vi "FindFilesNotRelativeToProjectRoot.vi"() -> ()   [LabVIEW 2020]
uses:
  <vilib>/Utility/lvfile.llb/NI_FileType.lvlib
  <vilib>/picture/picture.llb/imagedata.ctl
  <userlib>/_OpenG.lib/file/file.llb/openg_file.lvlib
  <userlib>/_OpenG.lib/file/file.llb/Valid Path - Traditional__ogtk.vi
  Microsoft.VisualBasic
panel:
  in  "Project":u16(ring)
  in  "Files Not in Project":i32[](listbox) caption="Files Not in Project (these files are on disk under the top-level project folder, but do not exist anywhere within the project)"
  in  "Move Files":bool
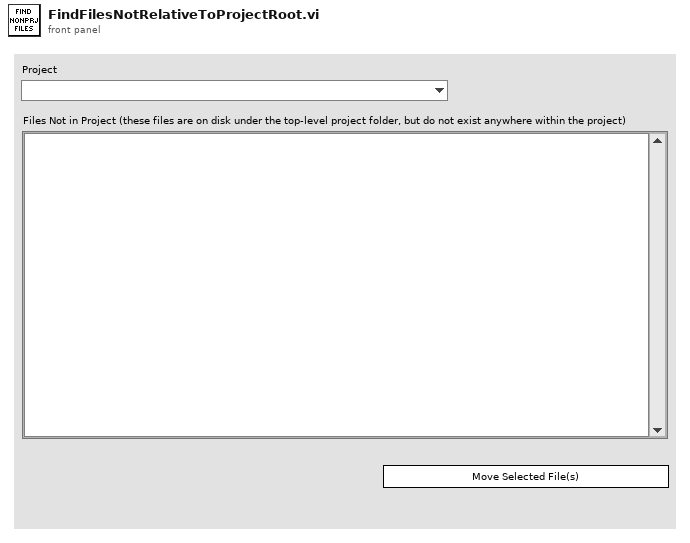
[diagram p1: front panel]
types:
  T1 = enum8{"Enabled", "Disabled", "Disabled and Grayed Out"}
  T2 = typedef "imagedata.ctl" = cluster{"image type":i32, "image depth":i32, "image":u8[], "mask":u8[], "colors":u32[], "Rectangle":cluster{"left":i16, "top":i16, "right":i16, "bottom":i16}}
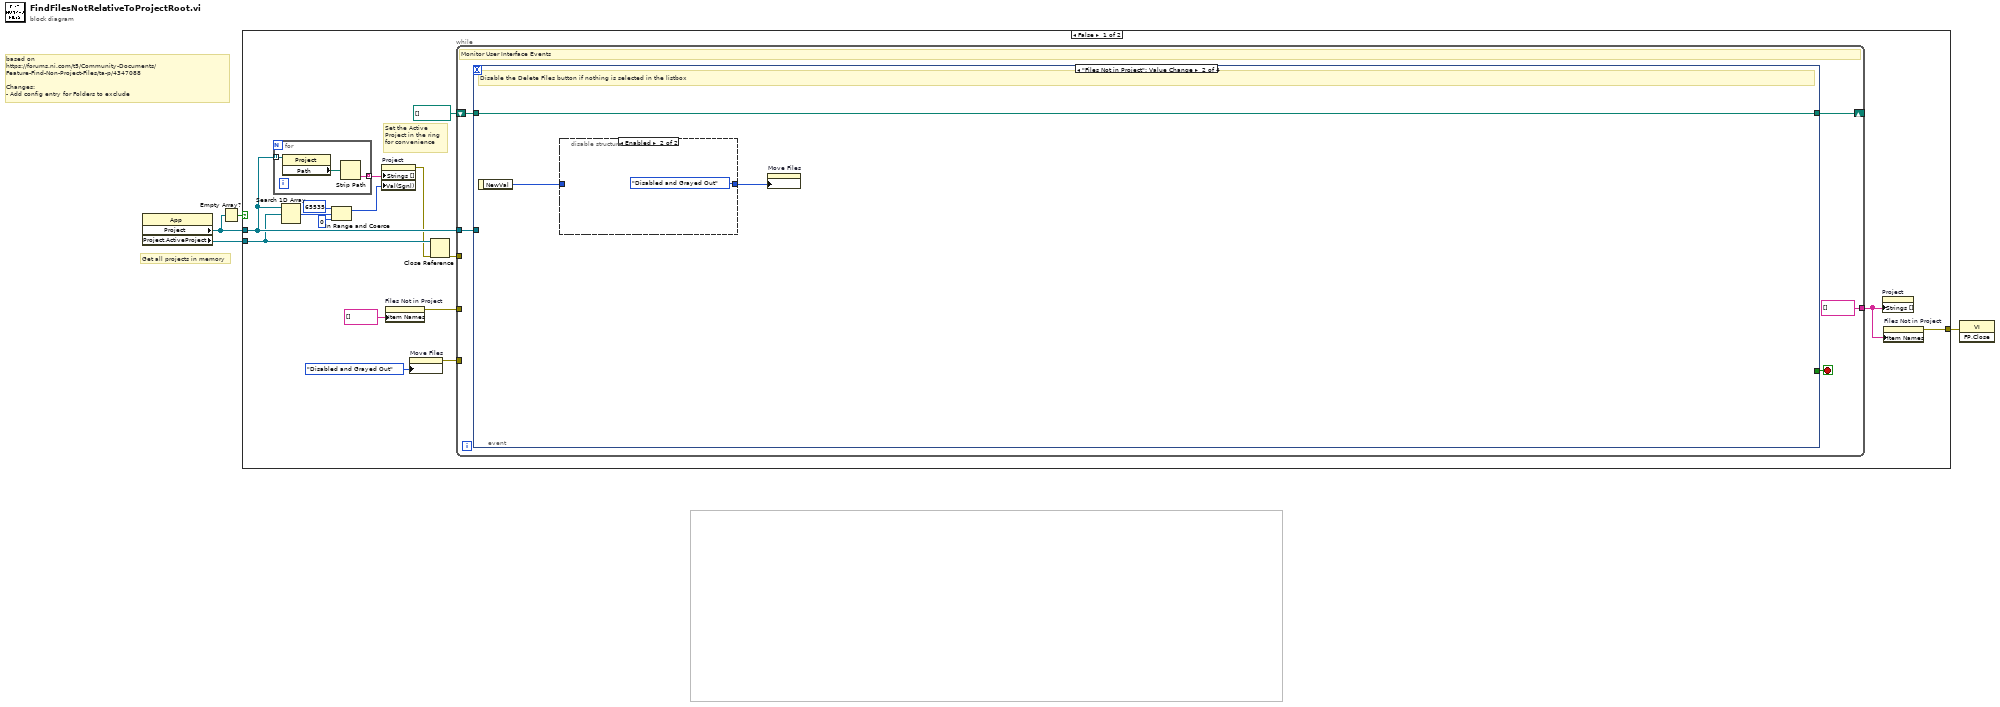
[diagram p0: block diagram]
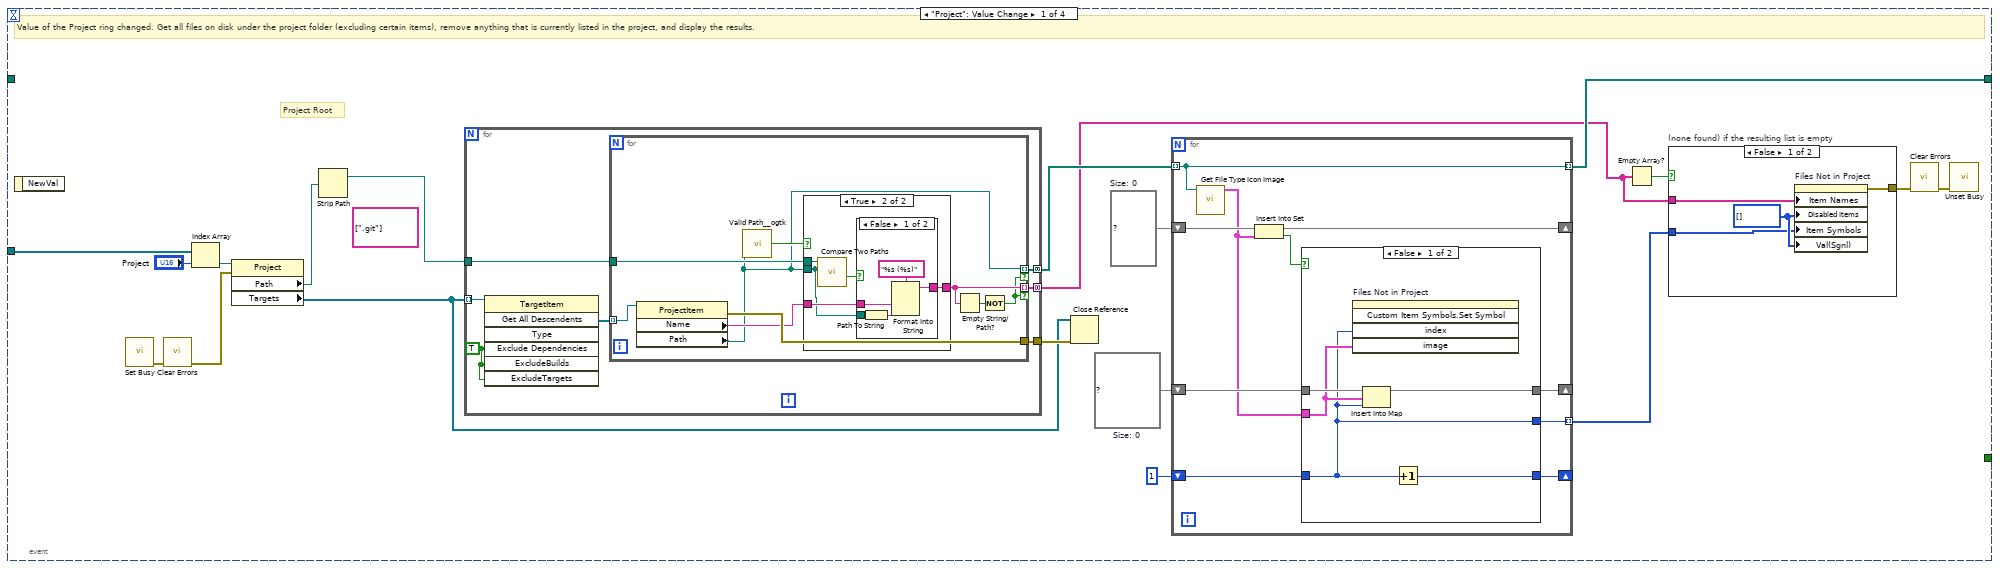
[diagram p2: hidden frame]
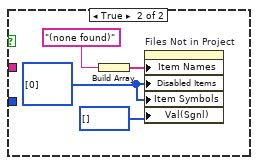
[diagram p3: hidden frame]
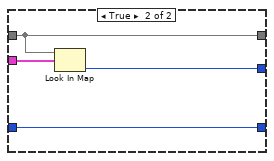
[diagram p6: hidden frame]
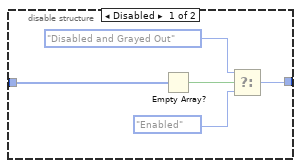
[diagram p7: hidden frame]
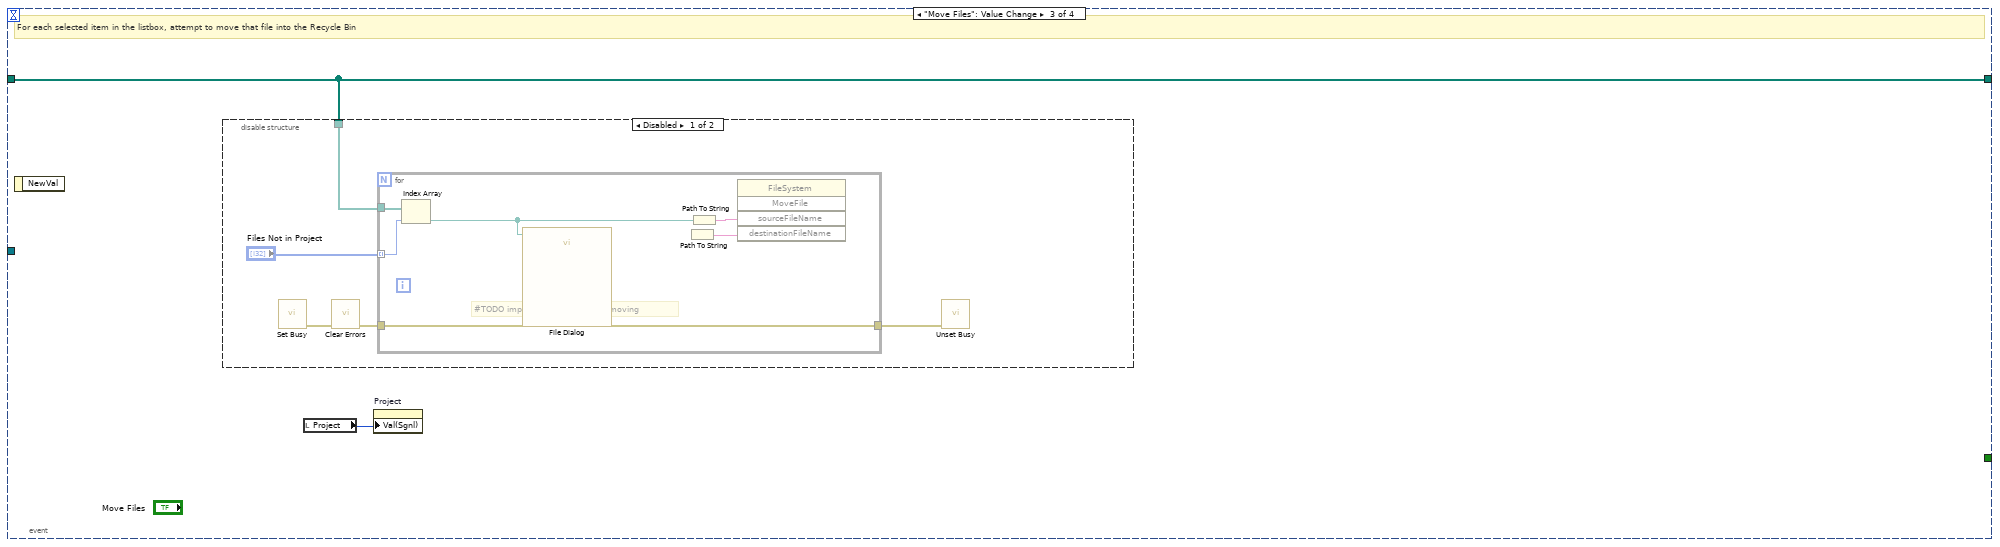
[diagram p8: hidden frame]
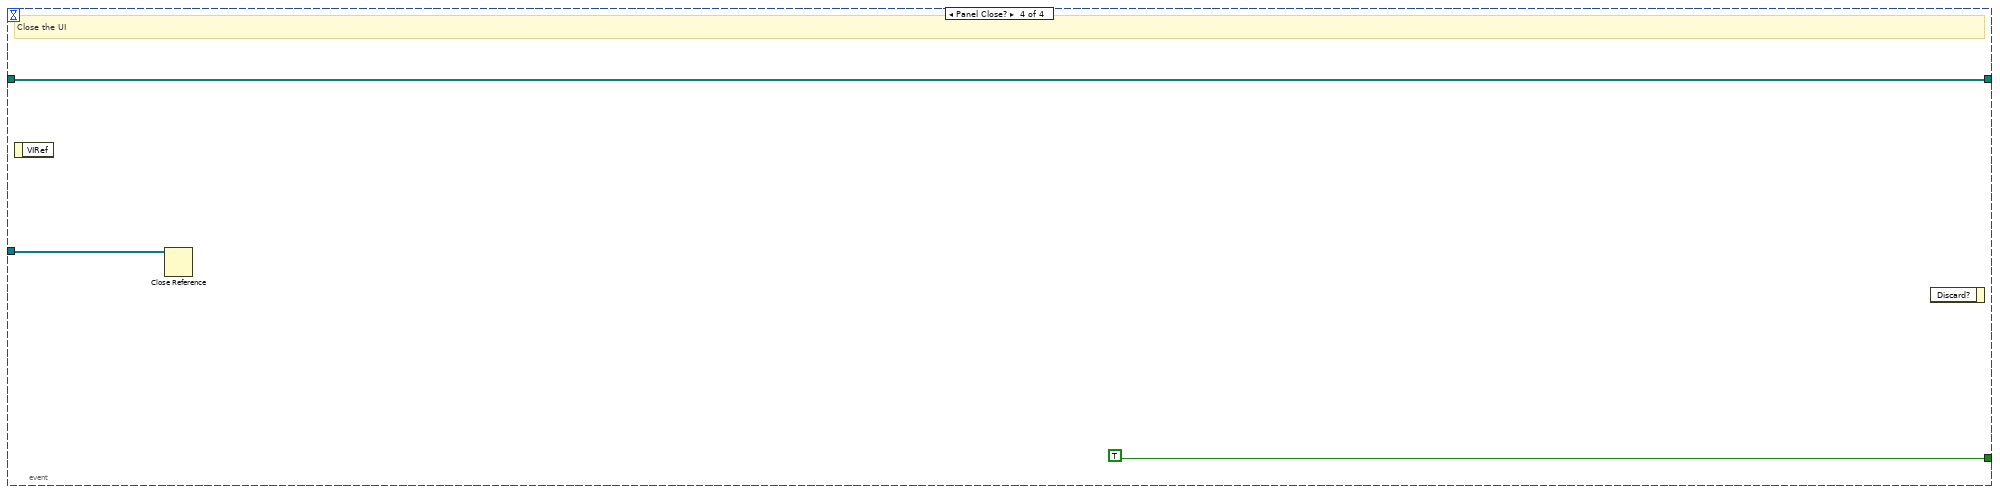
[diagram p10: hidden frame]
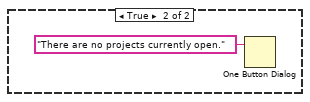
[diagram p11: hidden frame]
diagram:
  # "based on\nhttps://forums.ni.com/t5/Community-Documents/Feature-Find-Non-Project-Files/ta-p/4347088\n\nChanges:\n- Add config entry for Folders to exclude"
  # "Get all projects in memory"
  n1 = property class="App"() -> ("Project"=w3:refnum<vi>[], "Project.ActiveProject"=w4:refnum<vi>)  [unwired: 2 in, 2 out]
  n2 = Empty Array?(array=w3) -> (empty?=w2:bool)
  n3 = case shown="False" w2 {
    tunnel: w3 -> [w18 _]
    tunnel: w4 -> [w17 _]
    tunnel: [w9 _] -> w1
    frame False {
      # "Set the Active Project in the ring for convenience"
      n4 = for {
        tunnel: w18 -> [w23] mode=indexing
        tunnel: [w21] -> w19 mode=indexing
        n5 = property class="Project"(reference=w23) -> ("Path"=w22:path)  [unwired: 1 in, 2 out]
        n6 = Strip Path(path=w22) -> (name=w21:string)  [unwired: 1 out]
      }
      n7 = Search 1D Array(1D array=w18, element=w17) -> (index of element=w8:i32)  [unwired: 1 in]
      n8 = In Range and Coerce(upper limit=65535, x=w8, lower limit=0) -> (coerced(x)=w6:i32)  [unwired: 1 out]
      n9 = property on="Project" class="Ring (strict)"("Strings []"=w19, "Val(Sgnl)"=w6) -> (error out=w16:errorcluster)  [unwired: 2 in, 1 out]
      n10 = property on="Files Not in Project" class="LstBox (strict)"("Item Names"=string[] []) -> (error out=w12:errorcluster)  [unwired: 2 in, 1 out]
      n11 = property on="Move Files" class="Bool"("DisabledEnum"=T1."Disabled and Grayed Out" ("Disabled")) -> (error out=w13:errorcluster)  [unwired: 2 in, 1 out]
      n12 = Close Reference(reference=w17, error in (no error)=w16) -> (error out=w15:errorcluster)
      n13 = while {
        shift-right: [w28] -> _
        shift-left: path[] [] -> [w27]
        tunnel: w18 -> [w26]
        tunnel: w15 -> [_]
        tunnel: w13 -> [_]
        tunnel: w12 -> [_]
        tunnel: [string[] [] ("Strings []")] -> w10
        stop <- w25 stop-if-true
        # "Monitor User Interface Events"
        n14 = event shown="[1] \"Files Not in Project\": Value Change" {
          selector: _ -> [_ _ _ _]
          dyn-events: _ -> [_ _ _ _]
          timeout: _ -> [_ _ _ _]
          tunnel: [w46 w103 w111 w125] -> w28
          tunnel: w27 -> [_ w103 w111 w125]
          tunnel: w26 -> [w45 _ _ w123]
          tunnel: [_ _ _ TRUE ("Discard?")] -> w25
          event "Project": Value Change {
            w34 = set{T2} {}  # Size: 0
            w33 = map{T2, i32} {}  # Size: 0
            (unwired) string[] [".git"] ("Folders to Exclude")
            # "Project Root"
            # "Value of the Project ring changed. Get all files on disk under the project folder (excluding certain items), remove anything that is currently listed in the project, and display the results."
            n15 = event-data() -> ()  [unwired: 1 in, 1 out]
            n16 = call <vilib>:"Set Busy.vi"() -> ("error out"=w40:errorcluster)  [unwired: 10 in, 1 out]
            n17 = call <vilib>:"Clear Errors.vi"("error in (no error)"=w40) -> ("error out"=w39:errorcluster)  [unwired: 5 in, 1 out]
            n18 = Index Array(array=w45, index="Project") -> (element=w44:refnum<vi>)
            n19 = property class="Project"(reference=w44, error in=w39) -> ("Path"=w47:path, "Targets"=w41:refnum<vi>[])  [unwired: 2 out]
            n20 = Strip Path(path=w47) -> (stripped path=w31:path)  [unwired: 1 out]
            n21 = for {
              tunnel: w41 -> [w62] mode=indexing
              tunnel: [w60] -> w42
              tunnel: w31 -> [w59]
              tunnel: [w58] -> w29 mode=concatenating
              tunnel: [w57] -> w30 mode=concatenating
              w56 = TRUE ("ExcludeDependencies")
              n22 = invoke class="TargetItem" method="Get All Descendents"(reference=w62, "Exclude Dependencies"=w56, "ExcludeBuilds"=w56, "ExcludeTargets"=w56) -> ("All Descendents"=w61:refnum<vi>[])  [unwired: 3 in, 6 out]
              n23 = for {
                tunnel: w61 -> [w71] mode=indexing
                tunnel: [w69] -> w60
                tunnel: w59 -> [w70]
                tunnel: [w66] -> w58 mode=indexing if=w63
                tunnel: [w64] -> w57 mode=indexing if=w63
                n24 = property class="ProjectItem"(reference=w71) -> (error out=w69:errorcluster, "Name"=w67:string, "Path"=w64:path)  [unwired: 1 in, 1 out]
                n25 = call-poly <userlib>:"Valid Path__ogtk.vi"("path"=w64) -> ("valid"=w68:bool)
                n26 = case shown="True" w68 {
                  tunnel: w70 -> [_ w76]
                  tunnel: w64 -> [_ w73]
                  tunnel: w67 -> [_ w74]
                  tunnel: [_ w72] -> w66
                  frame False {
                  }
                  frame True {
                    n27 = call <vilib>:"Compare Two Paths.vi"("Path 2"=w73, "Path 1"=w76) -> ("Path 2 Relative to Path 1?"=w75:bool)  [unwired: 6 in, 3 out]
                    n28 = case shown="False" w75 {
                      tunnel: w74 -> [w80 _]
                      tunnel: w73 -> [w78 _]
                      tunnel: [w77 _] -> w72
                      frame False {
                        n29 = Path To String(path=w78) -> (string=w79:string)
                        n30 = Format Into String(format string="%s (%s)", w80, w79) -> (resulting string=w77:string)  [unwired: 2 in, 1 out]
                      }
                      frame True {
                      }
                    }
                  }
                }
                n31 = Empty String/Path?(string/path=w66) -> (empty?=w65:bool)
                n32 = Not(x=w65) -> (.not. x?=w63:bool)
              }
            }
            n33 = Close Reference(reference=w41, error in (no error)=w42) -> ()  [unwired: 1 out]
            n34 = for {
              tunnel: w30 -> [w91] mode=indexing
              tunnel: [w91] -> w46 mode=indexing
              shift-right: [w86] -> _
              shift-left: w34 -> [w87]
              shift-right: [w90] -> _
              shift-left: 1 -> [w89]
              shift-right: [w84] -> _
              shift-left: w33 -> [w88]
              tunnel: [w82] -> w32 mode=indexing
              n35 = call <vilib>:"Get File Type Icon Image.vi"("path"=w91) -> ("image data"=w83:T2)  [unwired: 9 in, 1 out]
              n36 = Insert Into Set(10:w83, 11:w87) -> (2:w85:bool, 3:w86:set{T2})
              n37 = case shown="False" w85 {
                tunnel: [w94 w100] -> w90
                tunnel: w89 -> [w92 w100]
                tunnel: w88 -> [w96 w99]
                tunnel: [w95 w99] -> w84
                tunnel: w83 -> [w93 w98]
                tunnel: [w92 w97] -> w82
                frame False {
                  n38 = invoke on="Files Not in Project" class="LstBox (strict)" method="Custom Item Symbols.Set Symbol"("index"=w92, "image"=w93) -> ()  [unwired: 3 in, 5 out]
                  n39 = Insert Into Map(map in=w96, key=w93, value=w92) -> (map out=w95:map{T2, i32})  [unwired: 2 out]
                  n40 = Increment(x=w92) -> (x+1=w94:i32)
                }
                frame True {
                  n41 = Look In Map(map=w99, key=w98) -> (value=w97:i32)  [unwired: 1 in, 1 out]
                }
              }
            }
            n42 = Empty Array?(array=w29) -> (empty?=w37:bool)
            n43 = case "(none found) if the resulting list is empty" shown="False" w37 {
              tunnel: w29 -> [w51 _]
              tunnel: [w49 _] -> w36
              tunnel: w32 -> [w48 _]
              frame False {
                w50 = i32[] [] ("Files")
                n44 = property on="Files Not in Project" class="LstBox (strict)"("Item Names"=w51, "Disabled Items"=w50, "Item Symbols"=w48, "Val(Sgnl)"=w50) -> (error out=w49:errorcluster)  [unwired: 2 in, 1 out]
              }
              frame True {
                w52 = i32[] [0] ("Files")
                n45 = Build Array("(none found)") -> (w55:string[])
                n46 = property on="Files Not in Project" class="LstBox (strict)"("Item Names"=w55, "Disabled Items"=w52, "Item Symbols"=w52, "Val(Sgnl)"=i32[] [] ("Files")) -> ()  [unwired: 2 in, 2 out]
              }
            }
            n47 = call <vilib>:"Clear Errors.vi"("error in (no error)"=w36) -> ("error out"=w38:errorcluster)  [unwired: 5 in, 1 out]
            n48 = call <vilib>:"Unset Busy.vi"("error in (no error)"=w38) -> ()  [unwired: 10 in, 1 out]
          }
          event "Files Not in Project": Value Change {
            # "Disable the Delete Files button if nothing is selected in the listbox"
            n49 = event-data() -> ("NewVal"=w102:i32[])  [unwired: 1 in]
            n50 = disable-structure shown="Enabled" {
              disable-tunnel: w102 -> [w108 _]
              disable-tunnel: [w106 T1."Disabled and Grayed Out" ("Disabled")] -> w101
              frame Disabled {
                n51 = Empty Array?(array=w108) -> (empty?=w107:bool)
                n52 = Select(t=T1."Disabled and Grayed Out" ("Disabled"), s=w107, f=T1."Enabled" ("Disabled")) -> (s? t:f=w106:T1)
              }
              frame Enabled {
              }
            }
            n53 = property on="Move Files" class="Bool"("DisabledEnum"=w101) -> ()  [unwired: 2 in, 2 out]
          }
          event "Move Files": Value Change {
            # "For each selected item in the listbox, attempt to move that file into the Recycle Bin"
            n54 = event-data() -> ()  [unwired: 1 in, 1 out]
            n55 = disable-structure shown="Disabled" {
              disable-tunnel: w111 -> [w116 _]
              frame Disabled {
                n56 = call <vilib>:"Set Busy.vi"() -> ("error out"=w114:errorcluster)  [unwired: 10 in, 1 out]
                n57 = call <vilib>:"Clear Errors.vi"("error in (no error)"=w114) -> ("error out"=w113:errorcluster)  [unwired: 5 in, 1 out]
                n58 = for {
                  tunnel: "Files Not in Project" -> [w121] mode=indexing
                  tunnel: w116 -> [w122]
                  tunnel: [w119] -> w112
                  tunnel: w113 -> [w119]
                  # "#TODO implement file dialog for moving"
                  n59 = Index Array(array=w122, index=w121) -> (element=w117:path)
                  n60 = call "File Dialog"("start path"=w117) -> ()  [unwired: 11 in, 4 out]
                  n61 = Path To String() -> (string=w118:string)  [unwired: 1 in]
                  n62 = Path To String(path=w117) -> (string=w120:string)
                  n63 = invoke class="FileSystem" method="MoveFile"("sourceFileName"=w120, "destinationFileName"=w118) -> ()  [unwired: 3 in, 5 out]
                }
                n64 = call <vilib>:"Unset Busy.vi"("error in (no error)"=w112) -> ()  [unwired: 10 in, 1 out]
              }
              frame Enabled {
              }
            }
            n65 = local read "Project"() -> (w110:u16)
            n66 = property on="Project" class="Ring (strict)"("Val(Sgnl)"=w110) -> ()  [unwired: 2 in, 2 out]
          }
          event Panel Close? {
            # "Close the UI"
            n67 = event-data() -> ()  [unwired: 1 in, 1 out]
            n68 = Close Reference(reference=w123) -> ()  [unwired: 1 in, 1 out]
            n69 = event-data() -> ()  [unwired: 2 in, 1 out]
          }
        }
      }
      n70 = property on="Project" class="Ring (strict)"("Strings []"=w10) -> ()  [unwired: 2 in, 2 out]
      n71 = property on="Files Not in Project" class="LstBox (strict)"("Item Names"=w10) -> (error out=w9:errorcluster)  [unwired: 2 in, 1 out]
    }
    frame True {
      n72 = One Button Dialog(message="There are no projects currently open.") -> ()  [unwired: 1 in, 1 out]
    }
  }
  n73 = invoke class="VI" method="FP.Close"(error in=w1) -> ()  [unwired: 2 in, 3 out]
